vi "part1.vi"() -> ()   [LabVIEW 2019]
panel:
  in  "Switch":bool
  in  "stop":bool
  out "LED":bool
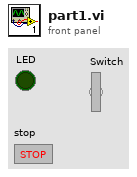
[diagram p1: front panel]
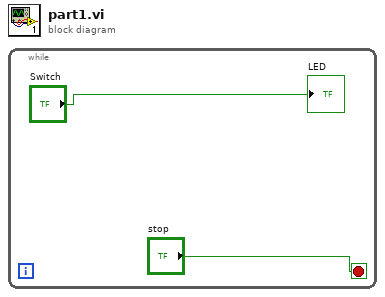
[diagram p0: block diagram]
diagram:
  n1 = while {
    stop <- "stop" stop-if-true
    "LED" <- "Switch"
  }
